vi "test_Series PID Simulated Scope Simualted FGen.vi"(8 "Error In":errorcluster) -> (0 "Error Out":errorcluster)   [LabVIEW 2023]
uses:
  Series/Series Base/Series Base.lvclass
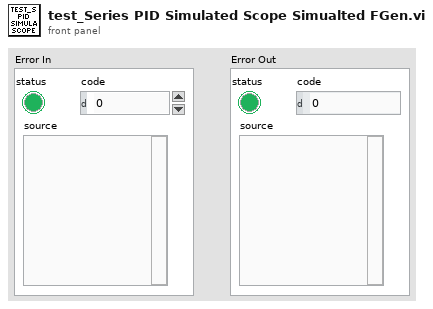
[diagram p1: front panel]
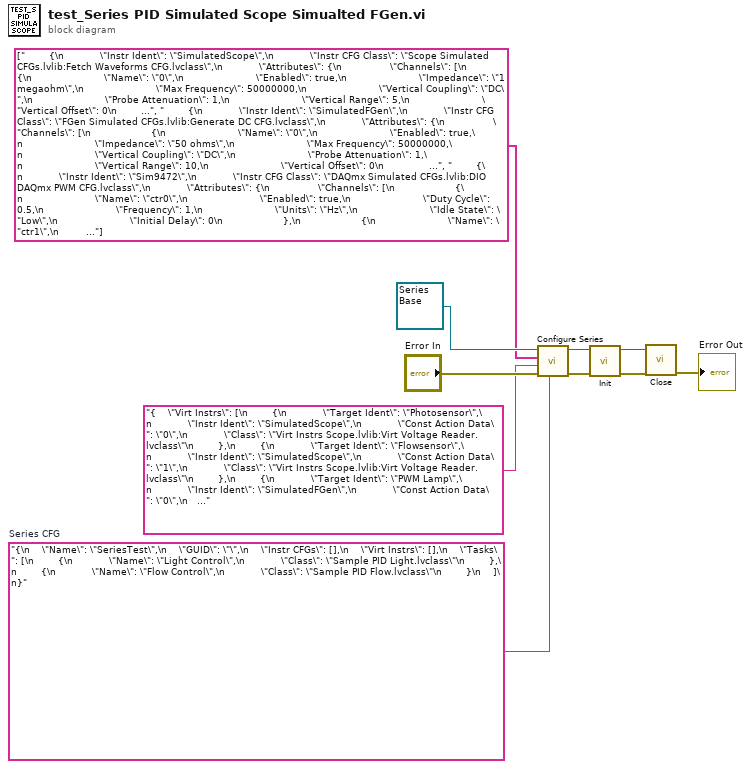
[diagram p0: block diagram]
diagram:
  w3 = "{\n    \"Name\": \"SeriesTest\",\n    \"GUID\": \"\",\n    \"Instr CFGs\": [],\n    \"Virt Instrs\": [],\n    \"Tasks\": [\n        {\n            \"Name\": \"Light Control\",\n            \"Class\": \"Sample PID Light.lvclass\"\n        },\n        {\n            \"Name\": \"Flow Control\",\n            \"Class\": \"Sample PID Flow.lvclass\"\n        }\n    ]\n}"  # Series CFG
  n1 = call "Configure Series.vi"("Series CFG"=w3, "error in (no error)"="Error In", "Virt Instrs CFG"="{    \"Virt Instrs\": [\n        {\n            \"Target Ident\": \"Photosensor\",\n            \"Instr Ident\": \"SimulatedScope\",\n            \"Const Action Data\": \"0\",\n            \"Class\": \"Virt Instrs Scope.lvlib:Virt Voltage Reader.lvclass\"\n        },\n        {\n            \"Target Ident\": \"Flowsensor\",\n            \"Instr Ident\": \"SimulatedScope\",\n            \"Const Action Data\": \"1\",\n            \"Class\": \"Virt Instrs Scope.lvlib:Virt Voltage Reader.lvclass\"\n        },\n        {\n            \"Target Ident\": \"PWM Lamp\",\n            \"Instr Ident\": \"SimulatedFGen\",\n            \"Const Action Data\": \"0\",\n            \"Class\": \"Virt Instrs FGen.lvlib:Virt Voltage Generator.lvclass\"\n        },\n        {\n            \"Target Ident\": \"PWM Flow\",\n            \"Instr Ident\": \"Sim9472\",\n            \"Const Action Data\": \"0\",\n            \"Class\": \"Virt Instrs DIO.lvlib:Virt PWM Generator.lvclass\"\n        }\n    ]\n}", "Instr CFGs"=string[] ["        {\n            \"Instr Ident\": \"SimulatedScope\",\n            \"Instr CFG Class\": \"Scope Simulated CFGs.lvlib:Fetch Waveforms CFG.lvclass\",\n            \"Attributes\": {\n                \"Channels\": [\n                    {\n                        \"Name\": \"0\",\n                        \"Enabled\": true,\n                        \"Impedance\": \"1 megaohm\",\n                        \"Max Frequency\": 50000000,\n                        \"Vertical Coupling\": \"DC\",\n                        \"Probe Attenuation\": 1,\n                        \"Vertical Range\": 5,\n                        \"Vertical Offset\": 0\n                    },\n                    {\n                        \"Name\": \"1\",\n                        \"Enabled\": true,\n                        \"Impedance\": \"50 ohms\",\n                        \"Max Frequency\": 50000000,\n                        \"Vertical Coupling\": \"DC\",\n                        \"Probe Attenuation\": 1,\n                        \"Vertical Range\": 5,\n                        \"Vertical Offset\": 0\n                    },\n                    {\n                        \"Name\": \"2\",\n                        \"Enabled\": false,\n                        \"Impedance\": \"50 ohms\",\n                        \"Max Frequency\": 50000000,\n                        \"Vertical Coupling\": \"DC\",\n                        \"Probe Attenuation\": 1,\n                        \"Vertical Range\": 5,\n                        \"Vertical Offset\": 0\n                    },\n                    {\n                        \"Name\": \"3\",\n                        \"Enabled\": false,\n                        \"Impedance\": \"50 ohms\",\n                        \"Max Frequency\": 50000000,\n                        \"Vertical Coupling\": \"DC\",\n                        \"Probe Attenuation\": 1,\n                        \"Vertical Range\": 1.4,\n                        \"Vertical Offset\": 0\n                    },\n                    {\n                        \"Name\": \"4\",\n                        \"Enabled\": false,\n                        \"Impedance\": \"50 ohms\",\n                        \"Max Frequency\": 50000000,\n                        \"Vertical Coupling\": \"DC\",\n                        \"Probe Attenuation\": 1,\n                        \"Vertical Range\": 5,\n                        \"Vertical Offset\": 0\n                    },\n                    {\n                        \"Name\": \"5\",\n                        \"Enabled\": false,\n                        \"Impedance\": \"50 ohms\",\n                        \"Max Frequency\": 50000000,\n                        \"Vertical Coupling\": \"DC\",\n                        \"Probe Attenuation\": 1,\n                        \"Vertical Range\": 5,\n                        \"Vertical Offset\": 0\n                    },\n                    {\n                        \"Name\": \"6\",\n                        \"Enabled\": false,\n                        \"Impedance\": \"50 ohms\",\n                        \"Max Frequency\": 50000000,\n                        \"Vertical Coupling\": \"DC\",\n                        \"Probe Attenuation\": 1,\n                        \"Vertical Range\": 5,\n                        \"Vertical Offset\": 0\n                    },\n                    {\n                        \"Name\": \"7\",\n                        \"Enabled\": false,\n                        \"Impedance\": \"50 ohms\",\n                        \"Max Frequency\": 50000000,\n                        \"Vertical Coupling\": \"DC\",\n                        \"Probe Attenuation\": 1,\n                        \"Vertical Range\": 5,\n                        \"Vertical Offset\": 0\n                    }\n                ],\n                \"Horizontal\": {\n                    \"Enforce Realtime\": true,\n                    \"Number of Records\": 1,\n                    \"Min Sample Rate\": 100000,\n                    \"Reference Position\": 50,\n                    \"Min Record Length\": 1000\n                },\n                \"Acquire\": {\n                    \"Type\": \"Normal\",\n                    \"NumSamples\": 1000,\n                    \"Fetch Relative To\": \"Read Pointer\"\n                },\n                \"Export Signal\": {\n                    \"Signal Identifier\": \"None\",\n                    \"Signal\": \"None\",\n                    \"Output Terminal\": \"None\"\n                },\n                \"Trigger\": {\n                    \"Type\": \"Immediate\",\n                    \"Slope\": \"Positive\",\n                    \"Source\": \"RTSI 0\",\n                    \"Holdoff\": 0,\n                    \"Delay\": 0\n                }\n            }\n        }", "        {\n            \"Instr Ident\": \"SimulatedFGen\",\n            \"Instr CFG Class\": \"FGen Simulated CFGs.lvlib:Generate DC CFG.lvclass\",\n            \"Attributes\": {\n                \"Channels\": [\n                    {\n                        \"Name\": \"0\",\n                        \"Enabled\": true,\n                        \"Impedance\": \"50 ohms\",\n                        \"Max Frequency\": 50000000,\n                        \"Vertical Coupling\": \"DC\",\n                        \"Probe Attenuation\": 1,\n                        \"Vertical Range\": 10,\n                        \"Vertical Offset\": 0\n                    },\n                    {\n                        \"Name\": \"1\",\n                        \"Enabled\": false,\n                        \"Impedance\": \"50 ohms\",\n                        \"Max Frequency\": 50000000,\n                        \"Vertical Coupling\": \"DC\",\n                        \"Probe Attenuation\": 1,\n                        \"Vertical Range\": 0.2,\n                        \"Vertical Offset\": 0\n                    }\n                ],\n                \"Horizontal\": {\n                    \"Enforce Realtime\": true,\n                    \"Number of Records\": 1,\n                    \"Min Sample Rate\": 100000,\n                    \"Reference Position\": 50,\n                    \"Min Record Length\": 1000\n                },\n                \"Acquire\": {\n                    \"Type\": \"Normal\"\n                },\n                \"Export Signal\": {\n                    \"Enabled\": false,\n                    \"Signal Identifier\": \"None\",\n                    \"Signal\": \"None\",\n                    \"Output Terminal\": \"None\"\n                },\n                \"Trigger\": {\n                    \"Type\": \"Digital\",\n                    \"Source\": \"RTSI 0\",\n                    \"Holdoff\": 0,\n                    \"Delay\": 0\n                }\n            }\n        }", "        {\n            \"Instr Ident\": \"Sim9472\",\n            \"Instr CFG Class\": \"DAQmx Simulated CFGs.lvlib:DIO DAQmx PWM CFG.lvclass\",\n            \"Attributes\": {\n                \"Channels\": [\n                    {\n                        \"Name\": \"ctr0\",\n                        \"Enabled\": true,\n                        \"Duty Cycle\": 0.5,\n                        \"Frequency\": 1,\n                        \"Units\": \"Hz\",\n                        \"Idle State\": \"Low\",\n                        \"Initial Delay\": 0\n                    },\n                    {\n                        \"Name\": \"ctr1\",\n                        \"Enabled\": false,\n                        \"Duty Cycle\": 0.5,\n                        \"Frequency\": 1,\n                        \"Units\": \"Hz\",\n                        \"Idle State\": \"Low\",\n                        \"Initial Delay\": 0\n                    },\n                    {\n                        \"Name\": \"ctr2\",\n                        \"Enabled\": false,\n                        \"Duty Cycle\": 0.5,\n                        \"Frequency\": 1,\n                        \"Units\": \"Hz\",\n                        \"Idle State\": \"Low\",\n                        \"Initial Delay\": 0\n                    },\n                    {\n                        \"Name\": \"ctr3\",\n                        \"Enabled\": false,\n                        \"Duty Cycle\": 0.5,\n                        \"Frequency\": 1,\n                        \"Units\": \"Hz\",\n                        \"Idle State\": \"Low\",\n                        \"Initial Delay\": 0\n                    }\n                ],\n                \"Timing\": {\n                    \"Samples per Channel\": 1000,\n                    \"Sample Mode\": \"Continuous Samples\",\n                    \"Sample Rate\": 0,\n                    \"Sample Clock Source\": \"Implicit\",\n                    \"Active Edge\": \"Rising\"\n                },\n                \"Trigger\": {\n                    \"Trigger Type\": \"No Trigger\"\n                }\n            }\n        }"], "HAL GOOP4:Series Base in"=refnum<class "Series Base.lvclass"> refnum ("HAL GOOP4.lvlib:Study Base.lvclass")) -> ("error out"=w6:errorcluster, "HAL GOOP4:Series Base out"=w7:refnum<class "Series Base.lvclass">)  [unwired: 5 in]
  n2 = call-dynamic "Init.vi"("error in (no error)"=w6, "HAL GOOP4:Series Base in"=w7) -> ("error out"=w10:errorcluster, "HAL GOOP4:Series Base out"=w9:refnum<class "Series Base.lvclass">)  [unwired: 8 in]
  n3 = call-dynamic "Close.vi"("error in (no error)"=w10, "HAL GOOP4:Series Base in"=w9) -> ("error out"=→"Error Out":errorcluster)  [unwired: 8 in, 1 out]
